vi "Plot Load maker V2 - scale.vi"(7 "Meta LUT":refnum<data-value>, 8 "error in (no error)":errorcluster, 11 "Scale reference":refnum<vi>) -> (0 "error out":errorcluster, 2 "Axis config":T1={"Name Label.Text"="", "Style"=0, "Tick Colors:Minor Tick Color"=0, "Tick Colors:Tick Color"=0, "Marker Colors:Text Color"=0, "Grid Colors:Major Color"=0, "Grid Colors:Minor Color"=0, "Mapping Mode"=0, "Flipped"=FALSE, "Name Label.Visible"=FALSE, "Name Label.Text Colors:Text Color"=0, "Scale Fit"=0, "Range:Maximum"=0.0, "Range:Minimum"=0.0, "Offset and Multiplier:Multiplier"=0.0, "Offset and Multiplier:Offset"=0.0, "Name Label.Font:Size"=0, "Marker.Font:Size"=0, "Uniform Marker Spacing?"=TRUE, "Format String"=""}, 3 "reference out":refnum<vi>)   [LabVIEW 2021, in "RocketPlot.lvlib"]
uses:
  RocketPlot.lvlib
  TypeDefs/Plot scale axis properties.ctl
  Plot scale refnum to LUT name.vi
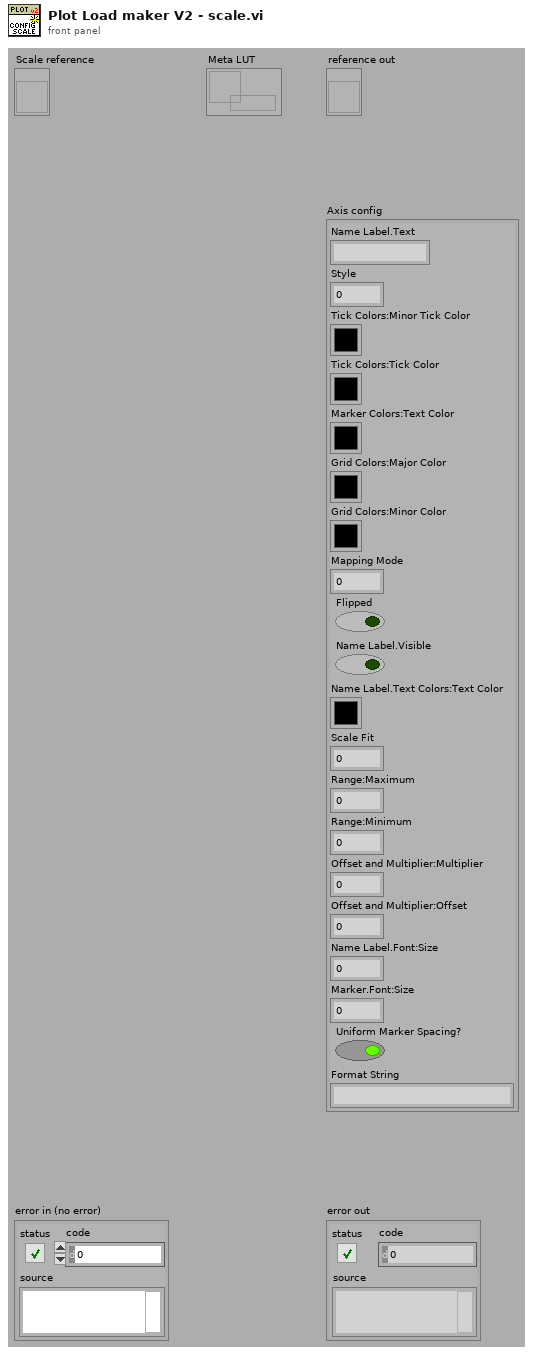
[diagram p1: front panel]
types:
  T1 = typedef "RocketPlot.lvlib/Plot scale axis properties.ctl" = cluster{"Name Label.Text":string, "Style":u8, "Tick Colors:Minor Tick Color":u32, "Tick Colors:Tick Color":u32, "Marker Colors:Text Color":u32, "Grid Colors:Major Color":u32, "Grid Colors:Minor Color":u32, "Mapping Mode":u8, "Flipped":bool, "Name Label.Visible":bool, "Name Label.Text Colors:Text Color":u32, "Scale Fit":u8, "Range:Maximum":dbl, "Range:Minimum":dbl, "Offset and Multiplier:Multiplier":dbl, "Offset and Multiplier:Offset":dbl, "Name Label.Font:Size":u32, "Marker.Font:Size":u32, "Uniform Marker Spacing?":bool, "Format String":string}
  T2 = typedef "RocketPlot.lvlib/Plot scale meta JSON.ctl" = cluster{"Type":T3, "Grid Colors:Major Color":u32, "Grid Colors:Minor Color":u32, "Style":u8, "Tick Colors:Tick Color":u32, "Tick Colors:Minor Tick Color":u32, "Format String":string, "State":T4, "AxisFocus":refnum<vi>}
  T3 = typedef "RocketPlot.lvlib/Plot axis.ctl" = enum16{"x axis", "left axis", "right axis"}
  T4 = typedef "RocketPlot.lvlib/Plot scale meta state.ctl" = cluster{"Visible":bool, "Focus":bool, "Multi-Y":bool}
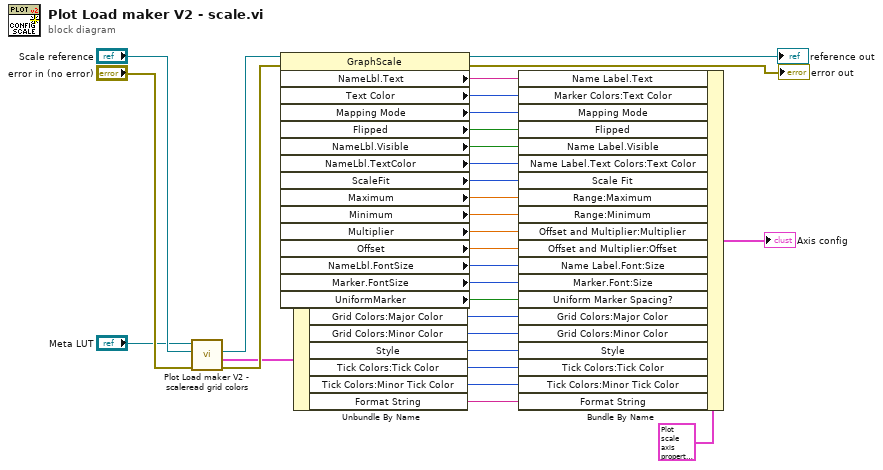
[diagram p0: block diagram]
diagram:
  n1 = call "Plot Load maker V2 - scaleread grid colors.vi"("error in (no error)"="error in (no error)", "Scale reference"="Scale reference", "Meta LUT"="Meta LUT") -> ("error out"=w7:errorcluster, "Scale LUT meta"=w1:T2, "Scale reference"=w8:refnum<vi>)  [unwired: 5 in, 1 out]
  n2 = property class="GraphScale"(reference=w8, error in=w7) -> (reference out=→"reference out":refnum<vi>, error out=→"error out":errorcluster, "NameLbl.Text"=w29:string, "Text Color"=w28:u32, "Mapping Mode"=w27:u8, "Flipped"=w26:bool, "NameLbl.Visible"=w25:bool, "NameLbl.TextColor"=w24:u32, "ScaleFit"=w23:u8, "Maximum"=w22:dbl, "Minimum"=w21:dbl, "Multiplier"=w20:dbl, "Offset"=w19:dbl, "NameLbl.FontSize"=w18:u32, "Marker.FontSize"=w17:u32, "UniformMarker"=w13:bool)
  n3 = Unbundle By Name(w1) -> ("Grid Colors:Major Color"=w12:u32, "Grid Colors:Minor Color"=w11:u32, "Style"=w6:u8, "Tick Colors:Tick Color"=w4:u32, "Tick Colors:Minor Tick Color"=w3:u32, "Format String"=w2:string)
  n4 = Bundle By Name(cluster=T1 {"Name Label.Text"="", "Style"=0, "Tick Colors:Minor Tick Color"=0, "Tick Colors:Tick Color"=0, "Marker Colors:Text Color"=0, "Grid Colors:Major Color"=0, "Grid Colors:Minor Color"=0, "Mapping Mode"=0, "Flipped"=FALSE, "Name Label.Visible"=FALSE, "Name Label.Text Colors:Text Color"=0, "Scale Fit"=0, "Range:Maximum"=0.0, "Range:Minimum"=0.0, "Offset and Multiplier:Multiplier"=0.0, "Offset and Multiplier:Offset"=0.0, "Name Label.Font:Size"=0, "Marker.Font:Size"=0, "Uniform Marker Spacing?"=TRUE, "Format String"=""} ("X-axis"), "Name Label.Text"=w29, "Marker Colors:Text Color"=w28, "Mapping Mode"=w27, "Flipped"=w26, "Name Label.Visible"=w25, "Name Label.Text Colors:Text Color"=w24, "Scale Fit"=w23, "Range:Maximum"=w22, "Range:Minimum"=w21, "Offset and Multiplier:Multiplier"=w20, "Offset and Multiplier:Offset"=w19, "Name Label.Font:Size"=w18, "Marker.Font:Size"=w17, "Uniform Marker Spacing?"=w13, "Grid Colors:Major Color"=w12, "Grid Colors:Minor Color"=w11, "Style"=w6, "Tick Colors:Tick Color"=w4, "Tick Colors:Minor Tick Color"=w3, "Format String"=w2) -> (→"Axis config":T1)
